vi "TimeTasker.vi"(4 "Last Que":dbl, 5 "Delay (sec)":dbl, 6 "Start Counting?":bool=TRUE, 7 "TeleOp Elapsed Seconds":dbl) -> (0 "Que":dbl, 2 "TimePast?":bool, 3 "TimePast":dbl)   [LabVIEW 2011]
uses:
  <vilib>/functionblocks/FB Core/FB Core.xnode
panel:
  out "elapsed time (ms)":i32
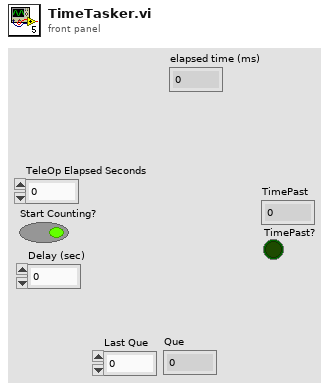
[diagram p1: front panel]
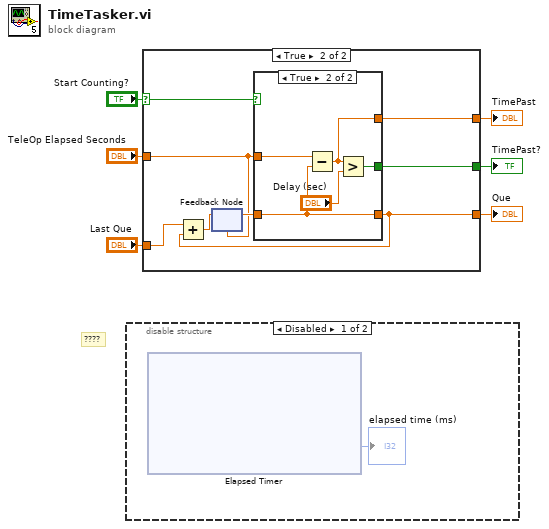
[diagram p0: block diagram]
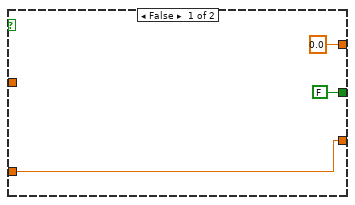
[diagram p3: hidden frame]
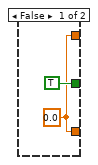
[diagram p4: hidden frame]
diagram:
  # "????"
  n1 = disable-structure shown="Disabled" {
    frame Disabled {
      n2 = xnode "Elapsed Timer"() -> ("elapsed time (ms)"=→"elapsed time (ms)":i32)  [unwired: 3 in, 1 out]
    }
    frame Enabled {
    }
  }
  n3 = case shown="True" "Start Counting?" {
    selector: "Start Counting?" -> [_ w14]
    tunnel: "TeleOp Elapsed Seconds" -> [_ w17]
    tunnel: [FALSE w16] -> w3
    tunnel: [0.0 ("TeleOp Elapsed Seconds") w15] -> w4
    tunnel: [w8 w12] -> w2
    tunnel: "Last Que" -> [w8 w13]
    frame False {
    }
    frame True {
      n4 = feedback #1(w17) -> (w18:dbl)
      n5 = case shown="True" w14 {
        tunnel: [w19 w24] -> w12
        tunnel: w18 -> [_ w24]
        tunnel: w17 -> [_ w25]
        tunnel: [TRUE w23] -> w16
        tunnel: [w19 w21] -> w15
        frame False {
          w19 = 0.0 ("TeleOp Elapsed Seconds")
        }
        frame True {
          n6 = Subtract(x=w25, y=w24) -> (x-y=w21:dbl)
          n7 = Greater?(x=w21, y="Delay (sec)") -> (0:w23:bool)
        }
      }
      n8 = Add(x=w13, y=w12) -> (x+y=w11:dbl)
      n9 = feedback-in #1(w11) -> ()
    }
  }
  "TimePast" <- w4
  "TimePast?" <- w3
  "Que" <- w2
